vi "Engine Init Test.vi"() -> ()   [LabVIEW 2019]
uses:
  Engine/Engine.lvclass
panel:
  out "Same Ref?":bool
  out "VersionString 2":string
  out "error out":errorcluster
  out "VersionString":string
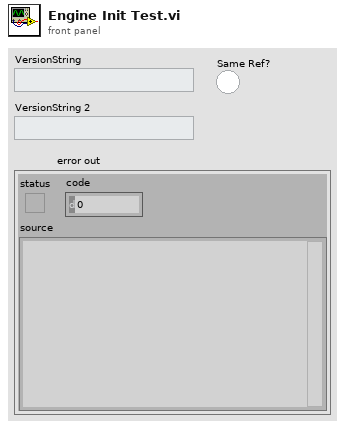
[diagram p1: front panel]
types:
  T1 = typedef "HTS.lvlib/Engine.lvclass/Session Handle.ctl" = refnum<data-value>
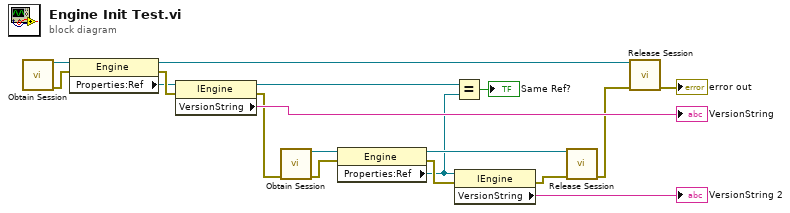
[diagram p0: block diagram]
diagram:
  n1 = call "Obtain Session.vi"() -> ("Session Handle"=w12:T1, "error out"=w11:errorcluster)  [unwired: 14 in]
  n2 = property class="Engine"(reference=w12, error in=w11) -> (reference out=w5:T1, error out=w17:errorcluster, "Properties:Ref"=w1:refnum<k7>)
  n3 = property class="IEngine"(reference=w1, error in=w17) -> (reference out=w14:refnum<k7>, error out=w10:errorcluster, "VersionString"=→"VersionString":string)
  n4 = call "Obtain Session.vi"("error in (no error)"=w10) -> ("Session Handle"=w9:T1, "error out"=w8:errorcluster)  [unwired: 13 in]
  n5 = property class="Engine"(reference=w9, error in=w8) -> (reference out=w7:T1, error out=w16:errorcluster, "Properties:Ref"=w2:refnum<k7>)
  n6 = Equal?(x=w14, y=w2) -> (x = y?=→"Same Ref?":bool)
  n7 = property class="IEngine"(reference=w2, error in=w16) -> (error out=w6:errorcluster, "VersionString"=→"VersionString 2":string)  [unwired: 1 out]
  n8 = call "Release Session.vi"("Session Handle"=w7, "error in (no error)"=w6) -> ("error out"=w4:errorcluster)  [unwired: 13 in]
  n9 = call "Release Session.vi"("Session Handle"=w5, "error in (no error)"=w4) -> ("error out"=→"error out":errorcluster)  [unwired: 13 in]
